vi "Logger Property Node.vi"   [LabVIEW 2017, in "Error Log.lvlib"]
doc: "Gets (reads) properties of an Error Logger. This node operates the same way as a standard Property Node. However, this node is pre-configured for Error Logger."
uses:
  Error Log.lvlib
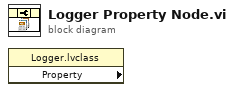
[diagram p0: block diagram]
diagram:
  n1 = property class="Logger.lvclass" props=[]() -> ()  [unwired: 2 in, 3 out]
